vi "DefaultFromINI.vi"(8 "error in (no error)":errorcluster, 11 "ChromaPowerSupplyModel":refnum<class "ChromaPowerSupplyModel.lvclass">) -> (0 "error out":errorcluster, 3 "ChromaPowerSupplyModel":refnum<class "ChromaPowerSupplyModel.lvclass">)   [LabVIEW 2018, in "AcPwrPlugins.lvlib" / "ChromaPowerSupplyModel.lvclass"]
doc: "This VI loads the instruments' configuration previously stored on file."
uses:
  ChromaPowerSupplyModel.lvclass
  C:/Program Files (x86)/National Instruments/LabVIEW 2018/user.lib/NIST/BaseClasses/BasePlugin_class/BasePlugin.lvclass
  C:/Projects/SmartGrid/ICDAS/NistPluggableModules/AcPwr/AcPwrPlugins/AcPwrBaseClass/AcPwrBase.lvclass
  ChromaPowerSupplyClass/TypeDefs/Device(s)Settings.ctl
  ChromaPowerSupplyClass/TypeDefs/Measurements.ctl
  TypeDefs/Database Settings.ctl
  <userlib>/NIST/BaseClasses/BasePlugin_class/BasePlugin.lvclass/BasePlugin.ctl
  <userlib>/NIST/BaseClasses/BasePlugin_class/Accessors/Read PluginIniFilePath.vi
  AcPwrBaseClass/AcPwrBase.lvclass
  ChromaPowerSupplyClass/ChromaPowerSupply.lvclass
  <vilib>/Utility/config.llb/NI_LVConfig.lvlib
  TestClass/Test.lvclass
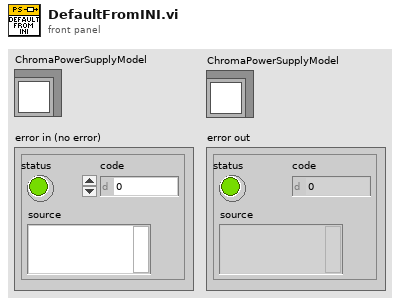
[diagram p1: front panel]
types:
  T1 = typedef "AcPwrPlugins.lvlib/ChromaPowerSupplyModel.lvclass/Database Settings.ctl" = cluster{"Data Source":string, "ICDAS to Model Table":string, "Model to ICDAS Table":string}
  T2 = typedef "AcPwrPlugins.lvlib/ChromaPowerSupply.lvclass/Measurements.ctl" = cluster{"Handle":string, "Name":string, "Enabled":bool, "Measurement Value":dbl, "btnMeasFetch":bool, "ProtectionStatusString":string, "Measurement Type":enum16{"Voltage", "Current", "Power"}}[]
  T3 = typedef "AcPwrPlugins.lvlib/ChromaPowerSupply.lvclass/Device(s)Settings.ctl" = cluster{"Phases":cluster{"Handle":string, "Instrument Options":string, "id query (T)":bool, "reset device (T)":bool, "Timing":cluster{"TimingOn":enum16{""}, "Hours":u32, "Minutes":u32, "Seconds":dbl, "CutoffVoltage":dbl}, "Connected":bool, "Output Mode":enum16{"Voltage (DC)", "Current (DC)"}, "Voltage":dbl, "Current":dbl, "Voltage Limit":dbl, "Current Limit":dbl, "Power Protect":dbl, "Current Protect":dbl, "Voltage Protect":dbl}[], "MeasName":string}
  T4 = typedef "Test.lvclass/INIInfo.ctl" = cluster{"Module Name":string, "INI File Name":string, "Class Name":string, "INI File Name Without Extension":string, "Module.Class.INI File Name":string, "Visualization VI Path":path, "Instrument Class Path":path}
  T5 = typedef "NI_LVConfig.lvlib/Config Data RefNum.ctl" = refnum<k1>
  T6 = cluster{"Device(s)Settings":T3, "Database Settings":T1}
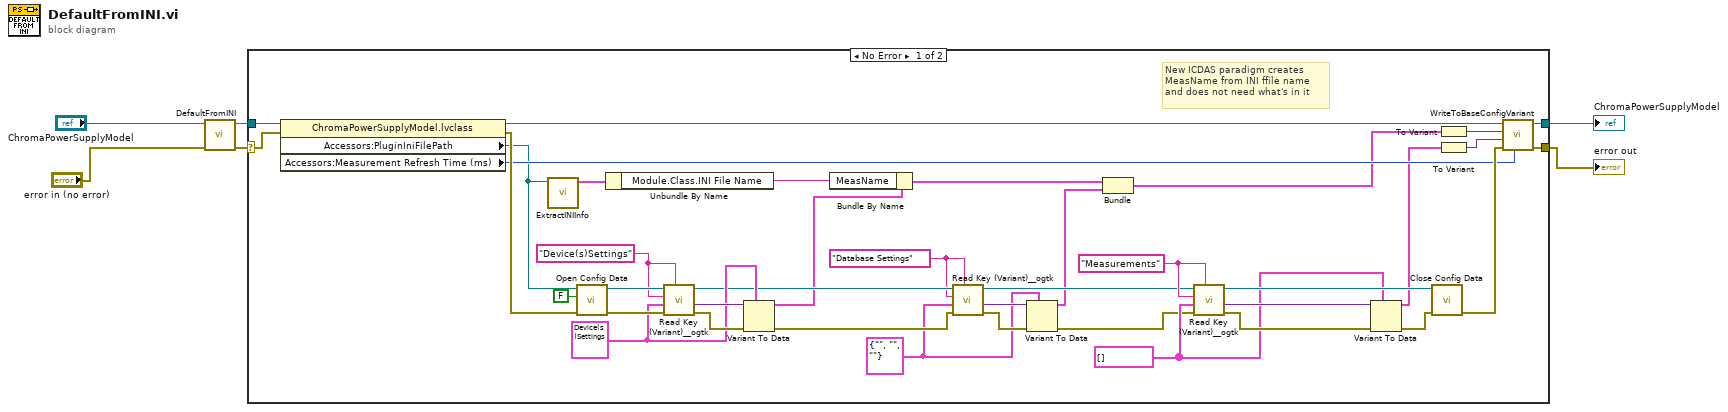
[diagram p0: block diagram]
diagram:
  n1 = call-parent "DefaultFromINI.vi"("error in (no error)"="error in (no error)", "AcPwrBase"="ChromaPowerSupplyModel") -> ("error out"=w6:errorcluster, "AcPwrBase"=w5:refnum<class "ChromaPowerSupplyModel.lvclass">)  [unwired: 8 in]
  n2 = case shown="No Error" w6 {
    selector: w6 -> [w37 w46]
    tunnel: w5 -> [w45 w47]
    tunnel: [w28 w47] -> w2
    tunnel: [w27 w46] -> w1
    frame No Error {
      w12 = "Database Settings" ("section")
      w11 = T1 {"Data Source"="", "ICDAS to Model Table"="", "Model to ICDAS Table"=""} ("Database Settings")
      w23 = T2 [] ("Measurements")
      w24 = T3 {"Phases"=[{"Handle"="", "Instrument Options"="", "id query (T)"=TRUE, "reset device (T)"=TRUE, "Timing"={"TimingOn"=enum."", "Hours"=0, "Minutes"=0, "Seconds"=0.0, "CutoffVoltage"=0.0}, "Connected"=FALSE, "Output Mode"=enum."Voltage (DC)", "Voltage"=0.0, "Current"=0.0, "Voltage Limit"=0.0, "Current Limit"=0.0, "Power Protect"=0.0, "Current Protect"=0.0, "Voltage Protect"=0.0}], "MeasName"=""} ("Device(s)Settings")
      w30 = "Measurements" ("section")
      w38 = "Device(s)Settings" ("section")
      # "New ICDAS paradigm creates\nMeasName from INI ffile name\nand does not need what's in it"
      n3 = property class="ChromaPowerSupplyModel.lvclass"(reference=w45, error in=w37) -> (reference out=w39:refnum<class "ChromaPowerSupplyModel.lvclass">, error out=w36:errorcluster, "Accessors:PluginIniFilePath"=w22:path, "Accessors:Measurement Refresh Time (ms)"=w26:u32)
      n4 = call "ExtractINIInfo.vi"("INI File Path"=w22) -> ("INI Info"=w20:T4)  [unwired: 8 in, 2 out]
      n5 = call <vilib>:"Open Config Data.vi"("error in (no error)"=w36, "create file if necessary (T)"=FALSE, "configuration file path"=w22) -> ("error out"=w42:errorcluster, "refnum"=w43:T5)  [unwired: 6 in, 1 out]
      n6 = Unbundle By Name(w20) -> ("Module.Class.INI File Name"=w19:string)
      n7 = call <userlib>:"Read Key (Variant)__ogtk.vi"("section"=w38, "error in (no error)"=w42, "type"=w24, "key (optional)"=w38, "refnum"=w43) -> ("error out"=w40:errorcluster, "key-value"=w41:variant, "refnum out"=w14:T5)  [unwired: 3 in, 1 out]
      n8 = Variant To Data(error in=w40, type=w24, Variant=w41) -> (data=w8:T3, error out=w16:errorcluster)
      n9 = Bundle By Name(cluster=w8, "MeasName"=w19) -> (w7:T3)
      n10 = call <userlib>:"Read Key (Variant)__ogtk.vi"("section"=w12, "error in (no error)"=w16, "type"=w11, "key (optional)"=w12, "refnum"=w14) -> ("error out"=w18:errorcluster, "key-value"=w17:variant, "refnum out"=w13:T5)  [unwired: 3 in, 1 out]
      n11 = Variant To Data(error in=w18, type=w11, Variant=w17) -> (data=w9:T1, error out=w15:errorcluster)
      n12 = Bundle("Device(s)Settings"=w7, "Database Settings"=w9) -> (w10:T6)  [unwired: 1 in]
      n13 = call <userlib>:"Read Key (Variant)__ogtk.vi"("section"=w30, "error in (no error)"=w15, "type"=w23, "key (optional)"=w30, "refnum"=w13) -> ("error out"=w34:errorcluster, "key-value"=w33:variant, "refnum out"=w32:T5)  [unwired: 3 in, 1 out]
      n14 = Variant To Data(error in=w34, type=w23, Variant=w33) -> (data=w21:T2, error out=w31:errorcluster)
      n15 = call <vilib>:"Close Config Data.vi"("error in (no error)"=w31, "refnum"=w32) -> ("error out"=w35:errorcluster)  [unwired: 8 in, 1 out]
      n16 = To Variant(anything=w10) -> (Variant=w29:variant)
      n17 = To Variant(anything=w21) -> (Variant=w25:variant)
      n18 = call-dynamic "WriteToBaseConfigVariant.vi"("Measurement Refresh Time (ms)"=w26, "error in (no error)"=w35, "Meas"=w25, "Config"=w29, "ChromaPowerSupplyModel in"=w39) -> ("error out"=w27:errorcluster, "ChromaPowerSupplyModel out"=w28:refnum<class "ChromaPowerSupplyModel.lvclass">)  [unwired: 5 in]
    }
    frame Error {
    }
  }
  "error out" <- w1
  "ChromaPowerSupplyModel" <- w2
